vi "AE Define.vi"(1 "error in":errorcluster) -> (0 "move?":bool, 4 "error out":errorcluster)   [LabVIEW 2013]
panel:
  out "?":T1(plugin-control)
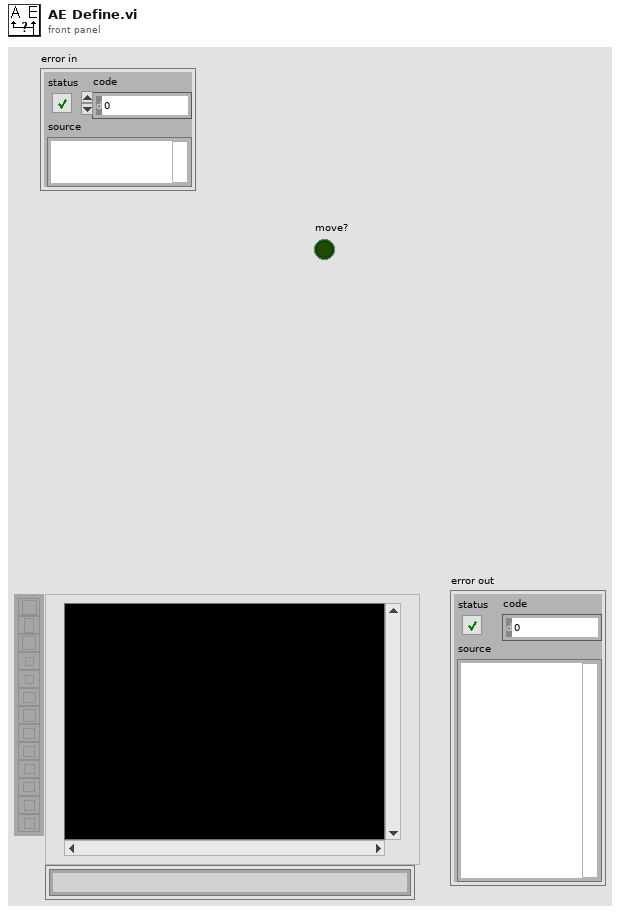
[diagram p1: front panel]
types:
  T1 = typedef "IMAQ Image.ctl" = refnum<image>
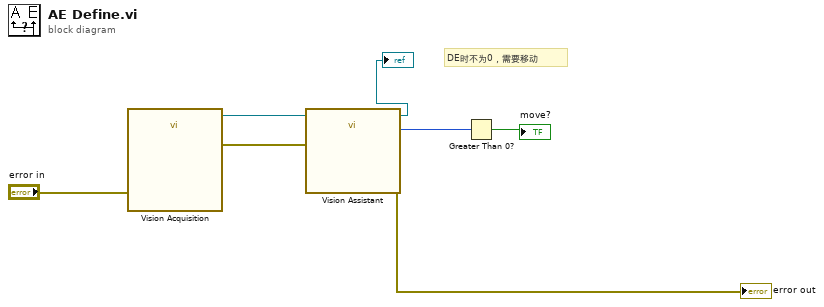
[diagram p0: block diagram]
diagram:
  # "DE时不为0，需要移动"
  n1 = call "Vision Acquisition"("error in"="error in") -> ("Image Out"=w6:T1, "error out"=w5:errorcluster)  [unwired: 25 in]
  n2 = call "Vision Assistant"("Image In"=w6, "error in"=w5) -> ("Image Out"=→"?":T1, "Number of Particles (Particle Analysis 1)"=w7:i32, "error out"=→"error out":errorcluster)  [unwired: 23 in]
  n3 = Greater Than 0?(x=w7) -> (x > 0?=→"move?":bool)
